vi "Test Print in Loop.vi"() -> ()   [LabVIEW 2014, in "Arduino SoftwareSerial Wrapper.lvlib"]
uses:
  Arduino SoftwareSerial Wrapper.lvlib
panel:
  out "Bytes written":u8
  out "Error Out":errorcluster
  in  "Error In":errorcluster
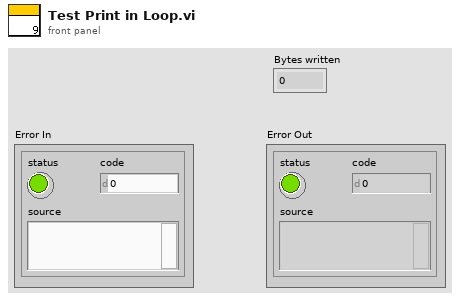
[diagram p1: front panel]
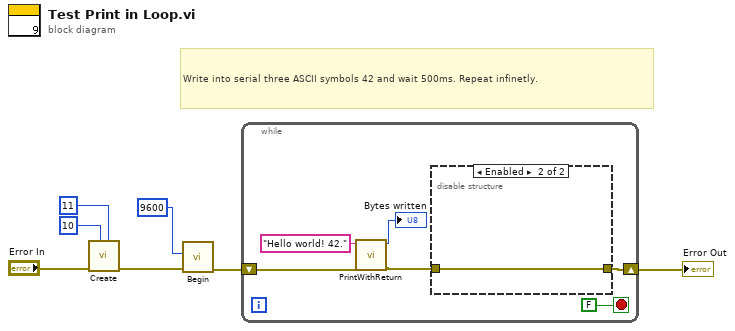
[diagram p0: block diagram]
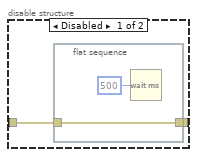
[diagram p2: hidden frame]
diagram:
  # "Write into serial three ASCII symbols 42 and wait 500ms. Repeat infinetly."
  n1 = call "Create.vi"("arduino RX pin"=u8 11 ("RX pin"), "arduino TX pin"=u8 10 ("RX pin"), "Error In"="Error In") -> ("Error Out"=w3:errorcluster)  [unwired: 8 in]
  n2 = call "Begin.vi"("Error In"=w3, "Baudrate"=u16 9600) -> ("Error Out"=w2:errorcluster)  [unwired: 8 in]
  n3 = while {
    shift-right: [w13] -> w4
    shift-left: w2 -> [w11]
    stop <- FALSE stop-if-true
    n4 = call "PrintWithReturn.vi"("Error In"=w11, "String to print"="Hello world! 42.") -> ("Error Out"=w10:errorcluster, "Bytes written"=→"Bytes written":u8)  [unwired: 8 in]
    n5 = disable-structure shown="Enabled" {
      disable-tunnel: [w15 w18] -> w13
      disable-tunnel: w10 -> [w14 w18]
      frame Disabled {
        n6 = flat-sequence {
          tunnel: [w16] -> w15
          tunnel: w14 -> [w16]
          frame #0 {
            n7 = Wait (ms)(milliseconds to wait=u32 500) -> ()  [unwired: 1 out]
          }
        }
      }
      frame Enabled {
      }
    }
  }
  "Error Out" <- w4
